vi "Day 8-Only Need 1 and 4.vi"() -> ()   [LabVIEW 2021]
uses:
  7a7e40d0-1107-41e4-9caf-784d51971341.vi
  52a580fe-a730-4ecf-827f-bdb76e2bd2ae.vi
  3dc89097-d59e-4e1c-8f80-55d6201ea7ec.vi
  6051aadd-e33c-4c9e-8f10-c58bb75e1c96.vi
  829ab1f4-53d9-4fed-a9bb-b7d095a32b7f.vi
  <vilib>/Utility/file.llb/Read Delimited Spreadsheet (string).vi
panel:
  out "Input":string[][](array[string])
  out "Solution":i64
  in  "Input File":enum32{"example input", "input"}(radio)
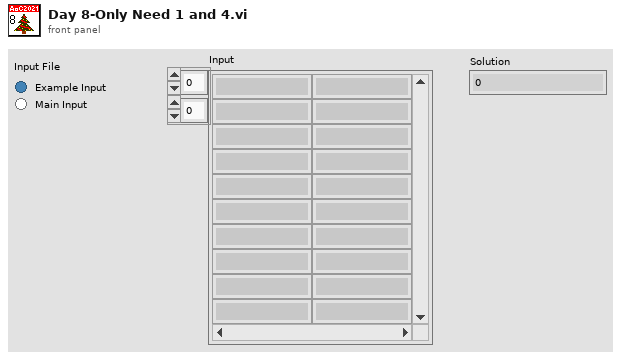
[diagram p1: front panel]
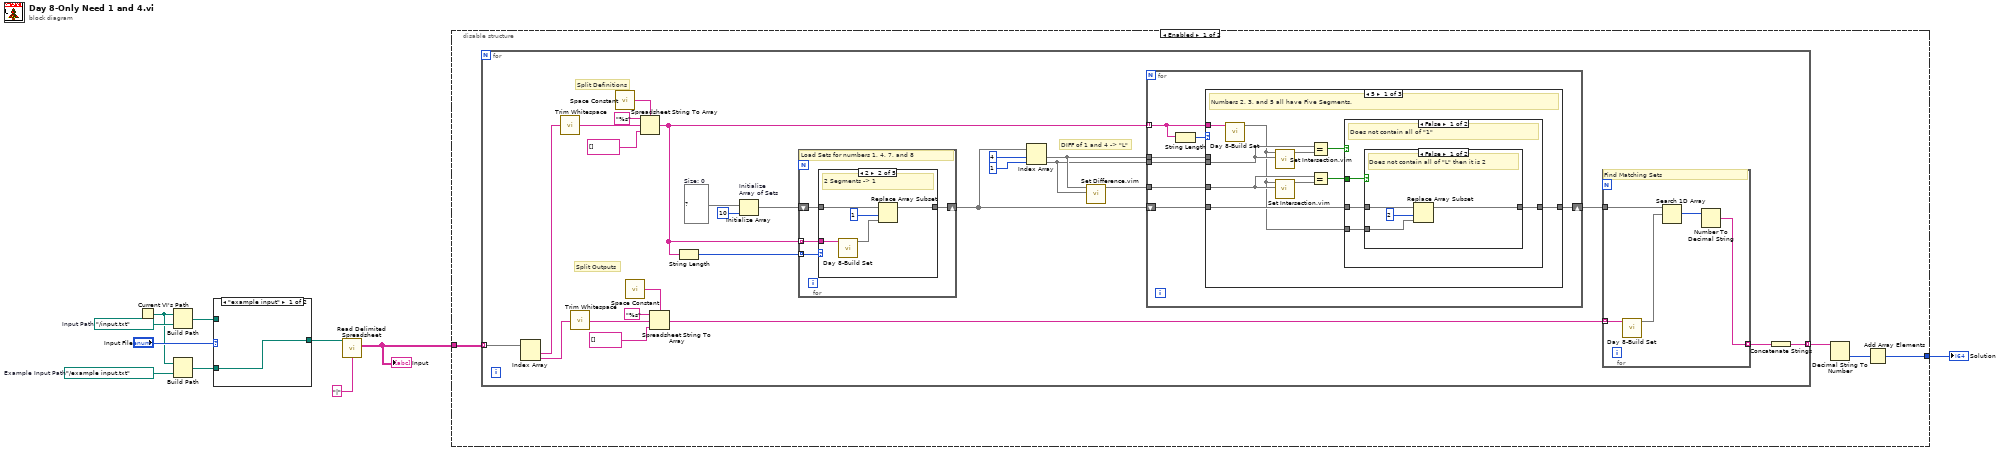
[diagram p0: block diagram]
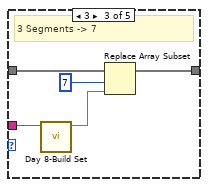
[diagram p3: hidden frame]
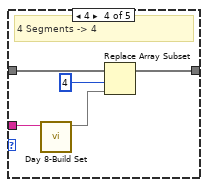
[diagram p4: hidden frame]
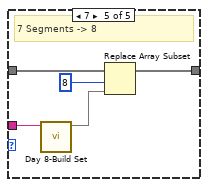
[diagram p5: hidden frame]
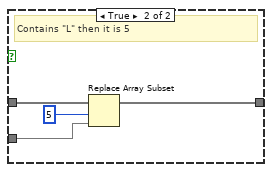
[diagram p6: hidden frame]
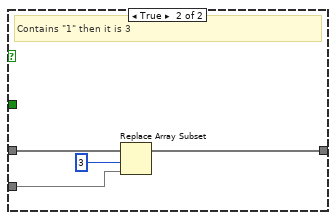
[diagram p7: hidden frame]
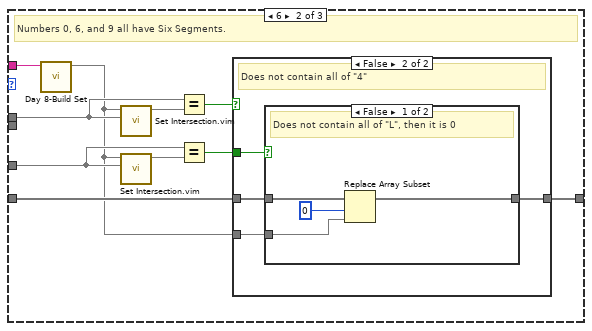
[diagram p8: hidden frame]
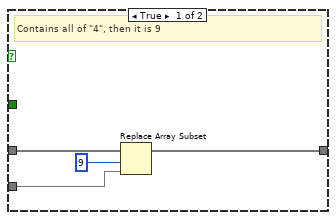
[diagram p9: hidden frame]
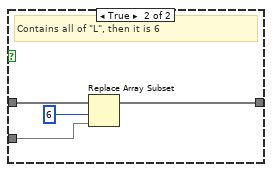
[diagram p10: hidden frame]
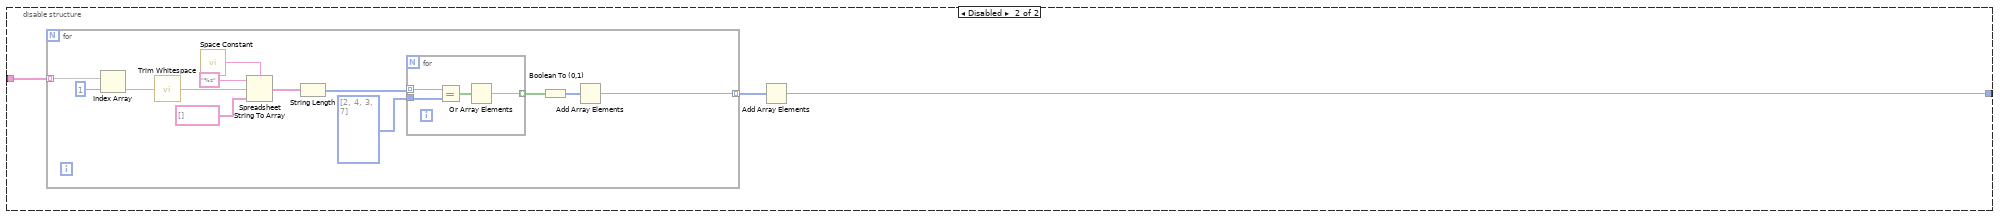
[diagram p12: hidden frame]
diagram:
  w9 = path "../example input.txt"  # Example Input Path
  w10 = path "../input.txt"  # Input Path
  n1 = Current VI's Path() -> (path=w4:path)
  n2 = Build Path(base path=w4, name or relative path=w10) -> (appended path=w7:path)
  n3 = Build Path(base path=w4, name or relative path=w9) -> (appended path=w6:path)
  n4 = case shown="\"example input\"" "Input File" {
    tunnel: w7 -> [_ w12]
    tunnel: w6 -> [w11 _]
    tunnel: [w11 w12] -> w5
    frame "example input" {
    }
    frame "input" {
    }
  }
  n5 = call-poly <vilib>:"Read Delimited Spreadsheet.vi"("file path (dialog if empty)"=w5, "delimiter (\\t)"="|" ("delimiter (\\t)")) -> ("all rows"=w1:string[][])  [unwired: 8 in, 5 out]
  "Input" <- w1
  n6 = disable-structure shown="Enabled" {
    disable-tunnel: w1 -> [w16 w135]
    disable-tunnel: [w15 w133] -> w3
    frame Enabled {
      n7 = for {
        tunnel: w16 -> [w41] mode=indexing
        tunnel: [w36] -> w14 mode=indexing
        w23 = set{string} {}  # Size: 0
        # "DIFF of 1 and 4 -> \"L\""
        # "Split Outputs"
        # "Split Definitions"
        n8 = Index Array(array=w41) -> (element #1=w31:string, element #2=w42:string)  [unwired: 2 in]
        n9 = call <vilib>:"Trim Whitespace.vi"("string"=w31) -> ("trimmed string"=w32:string)  [unwired: 1 in]
        n10 = call <vilib>:"Trim Whitespace.vi"("string"=w42) -> ("trimmed string"=w40:string)  [unwired: 1 in]
        n11 = call <vilib>:"Space Constant.vi"() -> ("String"=w35:string)
        n12 = call <vilib>:"Space Constant.vi"() -> ("String"=w37:string)
        n13 = Spreadsheet String To Array(delimiter (Tab)=w35, format string="%s", spreadsheet string=w32, array type (2D Dbl)=string[] []) -> (array=w27:string[])
        n14 = Spreadsheet String To Array(delimiter (Tab)=w37, format string="%s", spreadsheet string=w40, array type (2D Dbl)=string[] []) -> (array=w30:string[])
        n15 = String Length(string=w27) -> (length=w28:i32[])
        n16 = Initialize Array "Initialize\nArray of Sets"(w23, 10 ("dimension size")) -> (w25:set{string}[])
        n17 = for {
          tunnel: w28 -> [w46] mode=indexing
          tunnel: w27 -> [w45] mode=indexing
          shift-right: [w43] -> w20
          shift-left: w25 -> [w44]
          # "Load Sets for numbers 1, 4, 7, and 8"
          n18 = case shown="2" w46 {
            tunnel: w45 -> [_ w48 w54 w59 w64]
            tunnel: w44 -> [w47 w52 w57 w62 w67]
            tunnel: [w47 w49 w55 w60 w65] -> w43
            frame 0, Default {
            }
            frame 2 {
              # "2 Segments -> 1"
              n19 = call "Day 8-Build Set.vi"("String in"=w48) -> ("Set out"=w51:set{string})  [unwired: 10 in]
              n20 = Replace Array Subset(array=w52, new element=w51, index=1) -> (w49:set{string}[])
            }
            frame 3 {
              # "3 Segments -> 7"
              n21 = call "Day 8-Build Set.vi"("String in"=w54) -> ("Set out"=w53:set{string})  [unwired: 10 in]
              n22 = Replace Array Subset(array=w57, new element=w53, index=7) -> (w55:set{string}[])
            }
            frame 4 {
              # "4 Segments -> 4"
              n23 = call "Day 8-Build Set.vi"("String in"=w59) -> ("Set out"=w58:set{string})  [unwired: 10 in]
              n24 = Replace Array Subset(array=w62, new element=w58, index=4) -> (w60:set{string}[])
            }
            frame 7 {
              # "7 Segments -> 8"
              n25 = call "Day 8-Build Set.vi"("String in"=w64) -> ("Set out"=w63:set{string})  [unwired: 10 in]
              n26 = Replace Array Subset(array=w67, new element=w63, index=8) -> (w65:set{string}[])
            }
          }
        }
        n27 = Index Array(array=w20, index #1=4 ("index"), index #2=1 ("index")) -> (element #1=w18:set{string}, element #2=w17:set{string})
        n28 = call "Set Difference.vim"("set 2"=w17, "set 1"=w18) -> ("difference"=w19:set{string})  [unwired: 9 in]
        n29 = for {
          tunnel: w27 -> [w73] mode=indexing
          shift-right: [w71] -> w24
          shift-left: w20 -> [w72]
          tunnel: w18 -> [w70]
          tunnel: w19 -> [w69]
          tunnel: w17 -> [w68]
          n30 = String Length(string=w73) -> (length=w74:i32)
          n31 = case shown="5" w74 {
            tunnel: w73 -> [w76 w102 _]
            tunnel: w72 -> [w84 w110 w127]
            tunnel: [w83 w109 w127] -> w71
            tunnel: w70 -> [_ w107 _]
            tunnel: w69 -> [w77 w103 _]
            tunnel: w68 -> [w81 _ _]
            frame 5 {
              # "Numbers 2, 3, and 5 all have Five Segments."
              n32 = call "Day 8-Build Set.vi"("String in"=w76) -> ("Set out"=w75:set{string})  [unwired: 10 in]
              n33 = call "Set Intersection.vim"("set 2"=w81, "set 1"=w75) -> ("intersection"=w82:set{string})  [unwired: 9 in]
              n34 = call "Set Intersection.vim"("set 2"=w77, "set 1"=w75) -> ("intersection"=w79:set{string})  [unwired: 9 in]
              n35 = Equal?(x=w81, y=w82) -> (x = y?=w80:bool)
              n36 = Equal?(x=w77, y=w79) -> (x = y?=w78:bool)
              n37 = case shown="False" w80 {
                tunnel: w75 -> [w86 w97]
                tunnel: w84 -> [w88 w99]
                tunnel: [w87 w98] -> w83
                tunnel: w78 -> [w85 _]
                frame False {
                  # "Does not contain all of \"1\""
                  n38 = case shown="False" w85 {
                    tunnel: w88 -> [w91 w95]
                    tunnel: [w90 w94] -> w87
                    tunnel: w86 -> [w89 w93]
                    frame False {
                      # "Does not contain all of \"L\" then it is 2"
                      n39 = Replace Array Subset(array=w91, new element=w89, index=2) -> (w90:set{string}[])
                    }
                    frame True {
                      # "Contains \"L\" then it is 5"
                      n40 = Replace Array Subset(array=w95, new element=w93, index=5) -> (w94:set{string}[])
                    }
                  }
                }
                frame True {
                  # "Contains \"1\" then it is 3"
                  n41 = Replace Array Subset(array=w99, new element=w97, index=3) -> (w98:set{string}[])
                }
              }
            }
            frame 6 {
              # "Numbers 0, 6, and 9 all have Six Segments."
              n42 = call "Day 8-Build Set.vi"("String in"=w102) -> ("Set out"=w101:set{string})  [unwired: 10 in]
              n43 = call "Set Intersection.vim"("set 2"=w107, "set 1"=w101) -> ("intersection"=w108:set{string})  [unwired: 9 in]
              n44 = call "Set Intersection.vim"("set 2"=w103, "set 1"=w101) -> ("intersection"=w105:set{string})  [unwired: 9 in]
              n45 = Equal?(x=w107, y=w108) -> (x = y?=w106:bool)
              n46 = Equal?(x=w103, y=w105) -> (x = y?=w104:bool)
              n47 = case shown="False" w106 {
                tunnel: w101 -> [w111 w116]
                tunnel: w110 -> [w113 w118]
                tunnel: [w112 w117] -> w109
                tunnel: w104 -> [_ w115]
                frame True {
                  # "Contains all of \"4\", then it is 9"
                  n48 = Replace Array Subset(array=w113, new element=w111, index=9) -> (w112:set{string}[])
                }
                frame False {
                  # "Does not contain all of \"4\""
                  n49 = case shown="False" w115 {
                    tunnel: w118 -> [w121 w125]
                    tunnel: [w120 w124] -> w117
                    tunnel: w116 -> [w119 w123]
                    frame False {
                      # "Does not contain all of \"L\", then it is 0"
                      n50 = Replace Array Subset(array=w121, new element=w119, index=0) -> (w120:set{string}[])
                    }
                    frame True {
                      # "Contains all of \"L\", then it is 6"
                      n51 = Replace Array Subset(array=w125, new element=w123, index=6) -> (w124:set{string}[])
                    }
                  }
                }
              }
            }
            frame Default {
            }
          }
        }
        n52 = for {
          tunnel: w30 -> [w128] mode=indexing
          tunnel: [w130] -> w29 mode=indexing
          tunnel: w24 -> [w132]
          # "Find Matching Sets"
          n53 = call "Day 8-Build Set.vi"("String in"=w128) -> ("Set out"=w129:set{string})  [unwired: 10 in]
          n54 = Search 1D Array(1D array=w132, element=w129) -> (index of element=w131:i32)  [unwired: 1 in]
          n55 = Number To Decimal String(number=w131) -> (decimal integer string=w130:string)  [unwired: 1 in]
        }
        n56 = Concatenate Strings(w29) -> (w36:string)
      }
      n57 = Decimal String To Number(string=w14) -> (number=w13:i32[])  [unwired: 2 in, 1 out]
      n58 = Add Array Elements(numeric array=w13) -> (sum=w15:i32)
    }
    frame Disabled {
      n59 = for {
        tunnel: w135 -> [w146] mode=indexing
        tunnel: [w136] -> w134 mode=indexing
        n60 = Index Array(array=w146, index=1) -> (element=w147:string)
        n61 = call <vilib>:"Trim Whitespace.vi"("string"=w147) -> ("trimmed string"=w145:string)  [unwired: 1 in]
        n62 = call <vilib>:"Space Constant.vi"() -> ("String"=w142:string)
        n63 = Spreadsheet String To Array(delimiter (Tab)=w142, format string="%s", spreadsheet string=w145, array type (2D Dbl)=string[] []) -> (array=w141:string[])
        n64 = String Length(string=w141) -> (length=w140:i32[])
        n65 = for {
          tunnel: w140 -> [w152] mode=indexing
          tunnel: i32[] [2, 4, 3, 7] -> [w151]
          tunnel: [w149] -> w138 mode=indexing
          n66 = Equal?(x=w152, y=w151) -> (x = y?=w150:bool[])
          n67 = Or Array Elements(Boolean array=w150) -> (logical OR=w149:bool)
        }
        n68 = Boolean To (0,1)(Boolean=w138) -> (0, 1=w137:i16[])
        n69 = Add Array Elements(numeric array=w137) -> (sum=w136:i16)
      }
      n70 = Add Array Elements(numeric array=w134) -> (sum=w133:i16)
    }
  }
  "Solution" <- w3
